vi "Periodic Tasks.vi"(8 "error in":errorcluster) -> ()   [LabVIEW 2019]
doc: "This VI runs in parallel to other tasks. It can contain as many user-defined periodic loops as you need. These can carry out PID or other sorts of timed response."
uses:
  <vilib>/Rock Robotics/WPI/Utilities/WPI_GetSetVariantRefNum.vi
  Robot Global Data.vi
  <vilib>/Rock Robotics/Network Tables/NT Read Number.vi
  <vilib>/Rock Robotics/Network Tables/NT Write Number.vi
  <vilib>/Rock Robotics/Network Tables/NT Write Boolean.vi
  <vilib>/Rock Robotics/WPI/RobotDrive/WPI_RobotDriveArcadeDrive_Standard(NoSaturation).vi
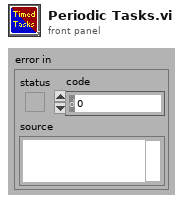
[diagram p1: front panel]
types:
  T1 = typedef "WPI_MotorControlDeviceRef.ctl" = cluster{"DeviceStatus":errorcluster, "Type":T2, "PWM":cluster{"PWM Channel":T3, "DeadBand":T4}, "CAN":cluster{"Device Number":u8, "SetOutput VI Ref":variant, "GetOutput VI Ref":variant, "Enable VI Ref":variant, "Disable VI Ref":variant, "Data":variant}, "Invert":bool, "DIO PWM":cluster{"PWM \"Enable\" Channel":T3, "DIOChannel":T5, "PWM Rate":dbl}}
  T2 = typedef "WPI_MotorControlType.ctl" = enum16{"PWM", "CAN", "DIO PWM"}
  T3 = typedef "FPGA_DIOPWMChannel.ctl" = enum8{"PWM 0", "PWM 1", "PWM 2", "PWM 3", "PWM 4", "PWM 5", "PWM 6", "PWM 7", "PWM 8", "PWM 9", "PWM MXP 0", "PWM MXP 1", "PWM MXP 2", "PWM MXP 3", "PWM MXP 4", "PWM MXP 5", "PWM MXP 6", "PWM MXP 7", "PWM MXP 8", "PWM MXP 9", "Invalid"}
  T4 = typedef "WPI_PWMDeadband.ctl" = cluster{"Name":string, "maxPositivePwm":i32, "minPositivePwm":i32, "centerPwm":i32, "maxNegativePwm":i32, "minNegativePwm":i32, "angularRange":u16}
  T5 = typedef "FPGA_DIOChannel.ctl" = enum8{"DIO 0", "DIO 1", "DIO 2", "DIO 3", "DIO 4", "DIO 5", "DIO 6", "DIO 7", "DIO 8", "DIO 9", "DIO MXP 0", "DIO MXP 1", "DIO MXP 2", "DIO MXP 3", "DIO MXP 4", "DIO MXP 5", "DIO MXP 6", "DIO MXP 7", "DIO MXP 8", "DIO MXP 9", "DIO MXP 10", "DIO MXP 11", "DIO MXP 12", "DIO MXP 13", "DIO MXP 14", "DIO MXP 15", "SPI Port CS1", "SPI Port CS2", "SPI Port CS3", "SPI Port MISO", "SPI Port MOSI", "Invalid"}
  T6 = typedef "WPI_JoystickDevRef.ctl" = cluster{"Device":T7}
  T7 = typedef "WPI_JoystickDeviceEnum.ctl" = enum16{"USB 0", "USB 1", "USB 2", "USB 3", "USB 4", "USB 5"}
  T8 = typedef "WPI_RobotDriveDevRef.ctl" = cluster{"DevStatus":errorcluster, "Motors[]":T1[], "Square Inputs":bool, "Max Output":dbl}
  T9 = cluster{"JoystickDevRef":T6, "RobotDriveDevRef":T8}
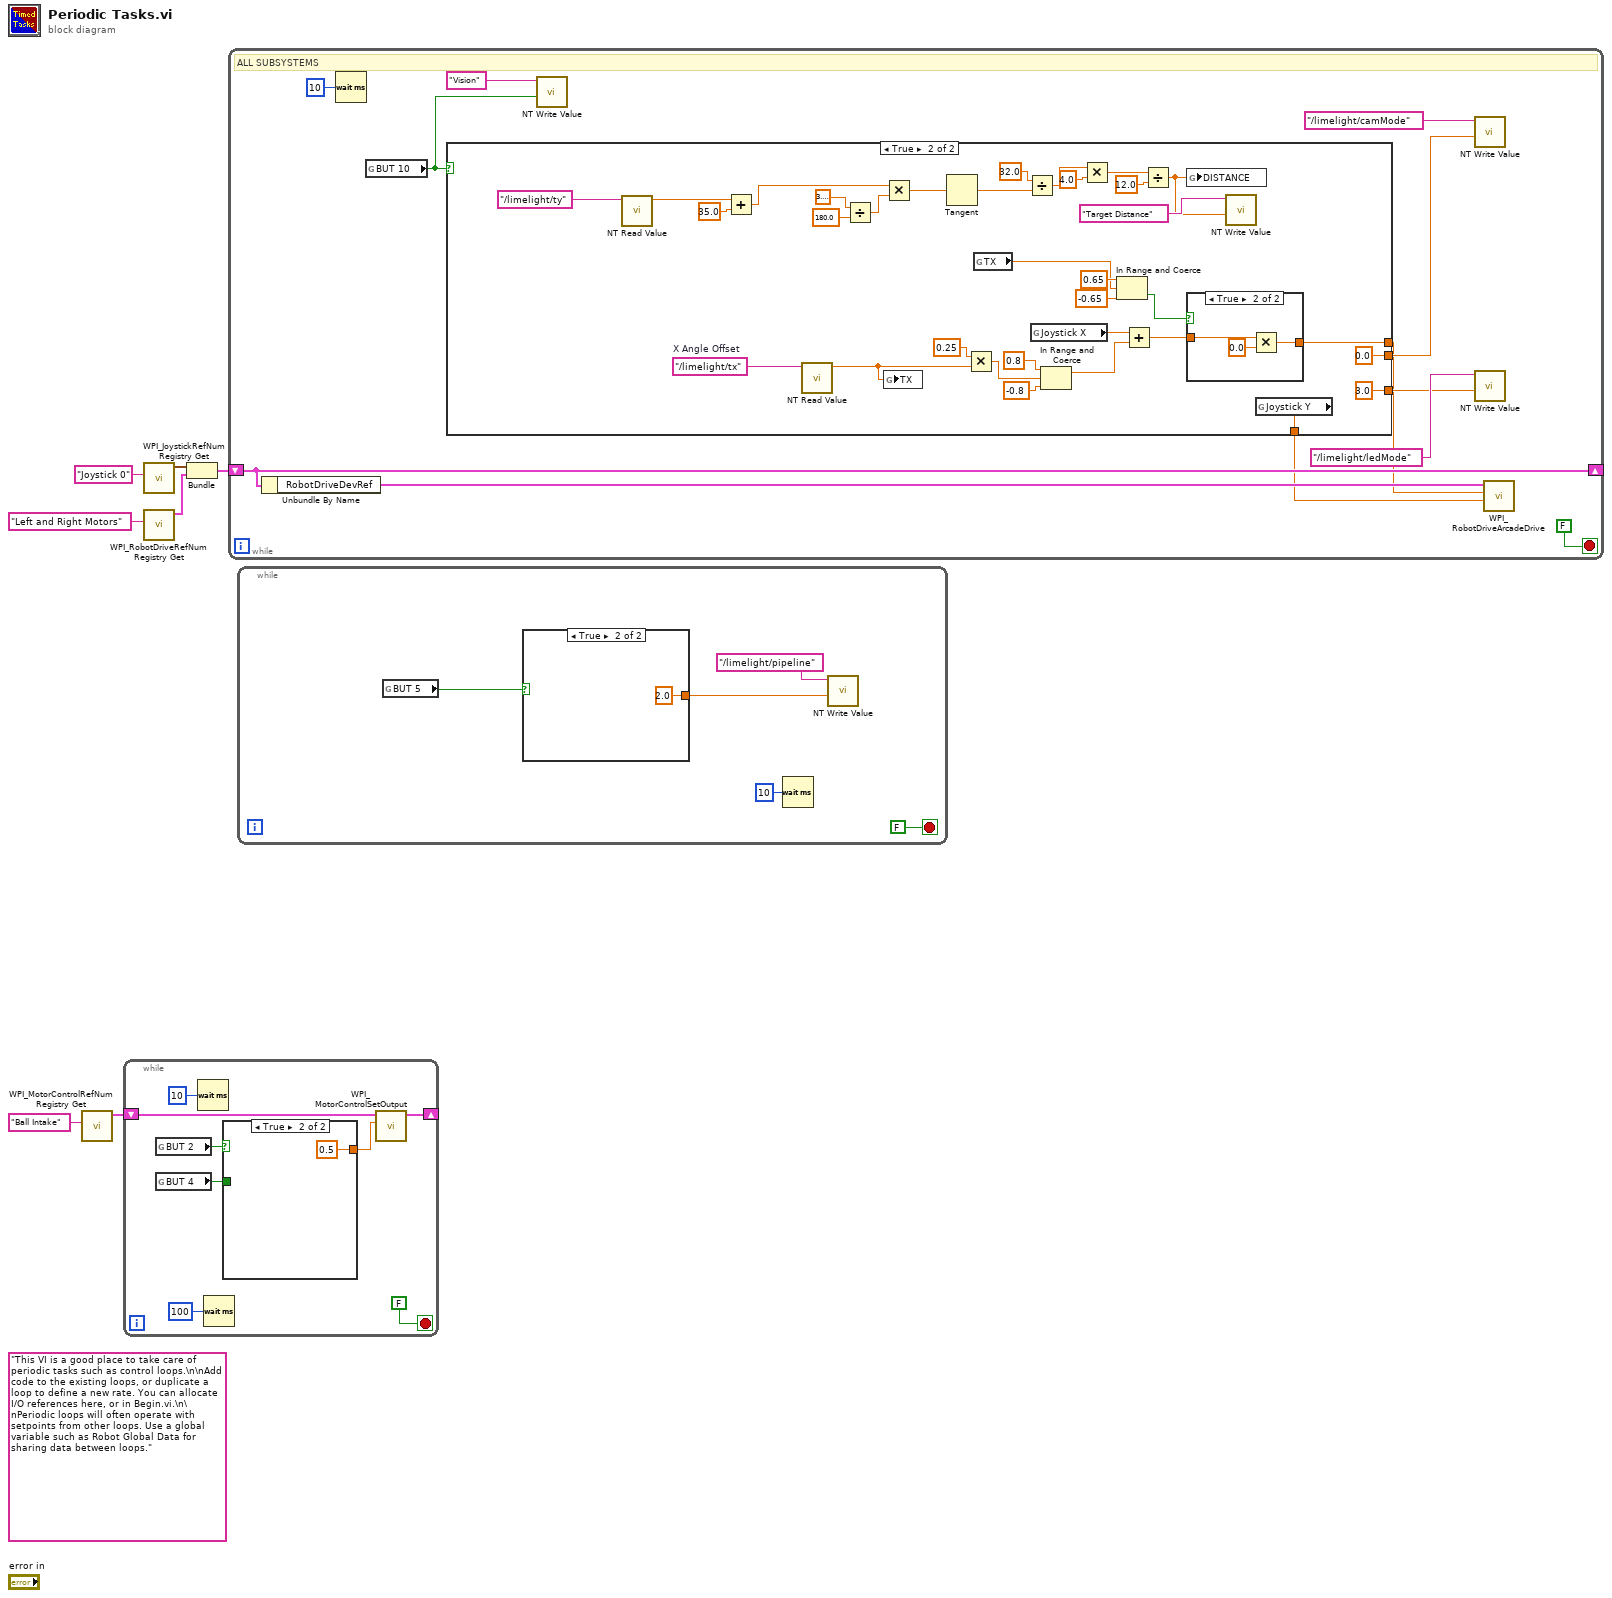
[diagram p0: block diagram]
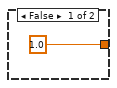
[diagram p2: hidden frame]
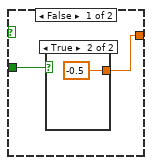
[diagram p3: hidden frame]
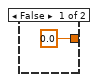
[diagram p4: hidden frame]
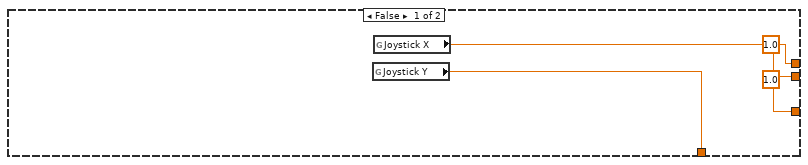
[diagram p5: hidden frame]
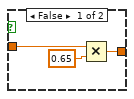
[diagram p6: hidden frame]
diagram:
  (unwired) "This VI is a good place to take care of periodic tasks such as control loops.\n\nAdd code to the existing loops, or duplicate a loop to define a new rate. You can allocate I/O references here, or in Begin.vi.\n\nPeriodic loops will often operate with setpoints from other loops. Use a global variable such as Robot Global Data for sharing data between loops."
  n1 = call <vilib>:"WPI_MotorControlRefNum Registry Get.vi"("refnum name"="Ball Intake") -> ("MotorControlDevRef"=w2:T1)  [unwired: 9 in, 1 out]
  n2 = while {
    shift-right: [w12] -> _
    shift-left: w2 -> [w11]
    stop <- FALSE stop-if-true
    n3 = global read "Robot Global Data.vi" "BUT 2"() -> (w14:bool)
    n4 = global read "Robot Global Data.vi" "BUT 4"() -> (w15:bool)
    n5 = Wait (ms)(milliseconds to wait=u32 10) -> ()  [unwired: 1 out]
    n6 = Wait (ms)(milliseconds to wait=u32 100) -> ()  [unwired: 1 out]
    n7 = case shown="True" w14 {
      tunnel: [w17 0.5 ("Output")] -> w13
      tunnel: w15 -> [w16 _]
      frame False {
        n8 = case shown="True" w16 {
          tunnel: [0.0 ("Output") -0.5 ("Output")] -> w17
          frame False {
          }
          frame True {
          }
        }
      }
      frame True {
      }
    }
    n9 = call <vilib>:"WPI_MotorControlSetOutput.vi"("Output"=w13, "MotorControlDevRef"=w11) -> ("MotorControlDevRef"=w12:T1)  [unwired: 7 in, 2 out]
  }
  n10 = call <vilib>:"WPI_JoystickRefNum Registry Get.vi"("refnum name"="Joystick 0") -> ("JoystickDevRef"=w5:T6)  [unwired: 1 in, 9 out]
  n11 = call <vilib>:"WPI_RobotDriveRefNum Registry Get.vi"("refnum name"="Left and Right Motors") -> ("RobotDriveDevRef"=w4:T8)  [unwired: 1 in, 9 out]
  n12 = Bundle("JoystickDevRef"=w5, "RobotDriveDevRef"=w4) -> (w3:T9)  [unwired: 1 out]
  n13 = while {
    shift-right: [w31] -> _
    shift-left: w3 -> [w31]
    stop <- FALSE stop-if-true
    # "ALL SUBSYSTEMS"
    n14 = Unbundle By Name(w31) -> ("RobotDriveDevRef"=w30:T8)
    n15 = Wait (ms)(milliseconds to wait=u32 10) -> ()  [unwired: 1 out]
    n16 = global read "Robot Global Data.vi" "BUT 10"() -> (w24:bool)
    n17 = case shown="True" w24 {
      tunnel: [1.0 ("Numeric") 0.0 ("Numeric")] -> w27
      tunnel: [1.0 ("Numeric") 3.0 ("Numeric")] -> w26
      tunnel: [w34 w42] -> w22
      tunnel: [w33 w41] -> w21
      frame False {
        n18 = global read "Robot Global Data.vi" "Joystick Y"() -> (w33:dbl)
        n19 = global read "Robot Global Data.vi" "Joystick X"() -> (w34:dbl)
      }
      frame True {
        w43 = "/limelight/tx"  # X Angle Offset
        n20 = call-poly <vilib>:"NT Read Value.vi"("Name"="/limelight/ty") -> ("Numeric"=w62:dbl)  [unwired: 9 in, 1 out]
        n21 = Add(x=w62, y=35.0) -> (x+y=w60:dbl)
        n22 = call-poly <vilib>:"NT Read Value.vi"("Name"=w43) -> ("Numeric"=w51:dbl)  [unwired: 9 in, 1 out]
        n23 = Divide(x=3.141592653589793, y=180.0) -> (x/y=w63:dbl)
        n24 = Multiply(x=w60, y=w63) -> (x*y=w59:dbl)
        n25 = global write "Robot Global Data.vi" "TX"(w51) -> ()
        n26 = Tangent(1:w59) -> (0:w69:dbl)
        n27 = Multiply(x=0.25 ("y"), y=w51) -> (x*y=w46:dbl)
        n28 = global read "Robot Global Data.vi" "TX"() -> (w37:dbl)
        n29 = Divide(x=32.0, y=w69) -> (x/y=w58:dbl)
        n30 = global read "Robot Global Data.vi" "Joystick X"() -> (w44:dbl)
        n31 = In Range and Coerce(upper limit=0.8, x=w46, lower limit=-0.8) -> (coerced(x)=w45:dbl)  [unwired: 1 out]
        n32 = Multiply(x=w58, y=4.0) -> (x*y=w56:dbl)
        n33 = In Range and Coerce(upper limit=0.65, x=w37, lower limit=-0.65) -> (In Range?=w40:bool)  [unwired: 1 out]
        n34 = Add(x=w44, y=w45) -> (x+y=w50:dbl)
        n35 = Divide(x=w56, y=12.0) -> (x/y=w52:dbl)
        n36 = global write "Robot Global Data.vi" "DISTANCE"(w52) -> ()
        n37 = case shown="True" w40 {
          tunnel: w50 -> [w71 w75]
          tunnel: [w72 w73] -> w42
          frame False {
            n38 = Multiply(x=w71, y=0.65) -> (x*y=w72:dbl)
          }
          frame True {
            n39 = Multiply(x=w75, y=0.0) -> (x*y=w73:dbl)
          }
        }
        n40 = call-poly <vilib>:"NT Write Value.vi"("Numeric"=w52, "Name"="Target Distance") -> ()  [unwired: 9 in, 1 out]
        n41 = global read "Robot Global Data.vi" "Joystick Y"() -> (w41:dbl)
      }
    }
    n42 = call-poly <vilib>:"NT Write Value.vi"("Boolean"=w24, "Name"="Vision") -> ()  [unwired: 9 in, 1 out]
    n43 = call-poly <vilib>:"NT Write Value.vi"("Numeric"=w27, "Name"="/limelight/camMode") -> ()  [unwired: 9 in, 1 out]
    n44 = call-poly <vilib>:"NT Write Value.vi"("Numeric"=w26, "Name"="/limelight/ledMode") -> ()  [unwired: 9 in, 1 out]
    n45 = call-poly <vilib>:"WPI_RobotDriveArcadeDrive.vi"("Y axis value"=w21, "X axis value"=w22, "RobotDriveDevRef"=w30) -> ()  [unwired: 6 in, 3 out]
  }
  n46 = while {
    stop <- FALSE stop-if-true
    n47 = global read "Robot Global Data.vi" "BUT 5"() -> (w77:bool)
    n48 = case shown="True" w77 {
      tunnel: [1.0 ("Default Value") 2.0 ("Default Value")] -> w76
      frame False {
      }
      frame True {
      }
    }
    n49 = Wait (ms)(milliseconds to wait=u32 10) -> ()  [unwired: 1 out]
    n50 = call-poly <vilib>:"NT Write Value.vi"("Numeric"=w76, "Name"="/limelight/pipeline") -> ()  [unwired: 9 in, 1 out]
  }
